vi "Set Shutter Ex.vi"(6 "extmode":i32, 7 "openingtime":i32, 9 "closingtime":i32, 10 "mode":i32, 11 "typ":i32) -> (3 "function return":u32)   [LabVIEW 2018, in "AndorSDK.lvlib"]
doc: "EXPNETTYPE unsigned int WINAPI SetShutterEx(int typ, int mode, int closingtime, int openingtime, int extmode);"
uses:
  AndorSDK.lvlib
  ATMCD32D.dll
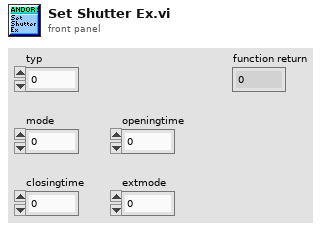
[diagram p1: front panel]
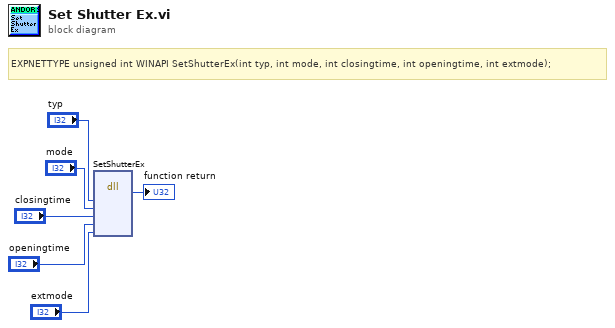
[diagram p0: block diagram]
diagram:
  # "EXPNETTYPE unsigned int WINAPI SetShutterEx(int typ, int mode, int closingtime, int openingtime, int extmode);"
  n1 = dll-call lib="PTH2babs E\nPersönliches02 - Arbeit03-HiwijobsLabviewCodelibANDOR\tAndor SDK\nATMCD32D.*" fn="SetShutterEx"("typ"="typ", "mode"="mode", "closingtime"="closingtime", "openingtime"="openingtime", "extmode"="extmode") -> (→"function return":u32)  [unwired: 8 in, 2 out]
